vi "获取关键参数.vi"(8 "error in (no error)":errorcluster caption="错误输入（无错误）", 9 "量程":u16, 10 "flowid":u16, 11 "id":i32) -> (0 "error out":errorcluster caption="错误输出")   [LabVIEW 2016, in "斯坦道总氮V2.lvlib"]
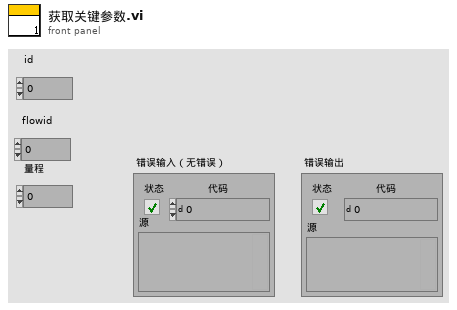
[diagram p1: front panel]
types:
  T1 = cluster{"运行模式":enum16{"维护模式", "常规模式", "应急模式", "质控模式"}, "质控频次":enum16{"关闭", "每天", "星期一", "星期二", "星期三", "星期四", "星期五", "星期六", "星期日"}, "空白核查时间":u16, "跨度核查时间":u16, "测量间隔":dbl}
  T2 = cluster{"标液浓度1":dbl, "测量吸光度1":dbl, "样品1启用":bool, "标液浓度2":dbl, "测量吸光度2":dbl, "样品2启用":bool, "标液浓度3":dbl, "测量吸光度3":dbl, "样品3启用":bool, "标液浓度4":dbl, "测量吸光度4":dbl, "样品4启用":bool, "标液浓度5":dbl, "测量吸光度5":dbl, "样品5启用":bool, "模型":enum32{"线性", "多项式"}, "精度":dbl, "XY图":cluster{"X Values":dbl[], "Y Values":dbl[]}[], "拟合公式":string, "r^2":dbl, "标样一校准时间":timestamp, "标样二校准时间":timestamp, "标样三校准时间":timestamp, "标样四校准时间":timestamp, "标样五校准时间":timestamp, "二次方程":cluster{"c":dbl, "x":dbl, "x^2":dbl}, "标定时间":timestamp}
  T3 = cluster{"精度":dbl, "检出限":dbl, "量程上限":dbl, "量程下限":dbl}
  T4 = cluster{"总磷":dbl, "总氮":dbl, "氨氮":dbl, "磷酸盐":dbl, "硝氮":dbl, "亚硝氮":dbl, "硅酸盐":dbl, "硫化物":dbl, "COD":dbl}
  T5 = cluster{"标液浓度1":dbl, "测量吸光度1":dbl, "样品1启用":bool, "标液浓度2":dbl, "测量吸光度2":dbl, "样品2启用":bool, "标液浓度3":dbl, "测量吸光度3":dbl, "样品3启用":bool, "标液浓度4":dbl, "测量吸光度4":dbl, "样品4启用":bool, "标液浓度5":dbl, "测量吸光度5":dbl, "样品5启用":bool, "模型":enum32{"线性", "多项式"}, "精度":dbl, "XY图":cluster{"X Values":dbl[], "Y Values":dbl[]}[], "拟合公式":string, "r^2":dbl, "标样一校准时间":timestamp, "标样二校准时间":timestamp, "标样三校准时间":timestamp, "标样四校准时间":timestamp, "标样五校准时间":timestamp, "二次方程":cluster{"c":dbl, "x":dbl, "x^2":dbl}, "标定时间":timestamp}[]
  T6 = typedef "斯坦道总氮V2.lvlib/关键参数.ctl" = cluster{"测量量程":sgl, "测量检出限":sgl, "测量精度":sgl, "测量间隔":sgl, "消解温度":sgl, "消解时长":sgl, "三项式系数":sgl, "二次多项式系数":sgl, "曲线斜率":sgl, "曲线截距":sgl, "线性相关系数":sgl, "空白校准时间":timestamp, "标样校准时间":timestamp, "测量信号值":sgl, "稀释倍数":sgl, "空白标定系数":sgl, "量程系数":sgl}
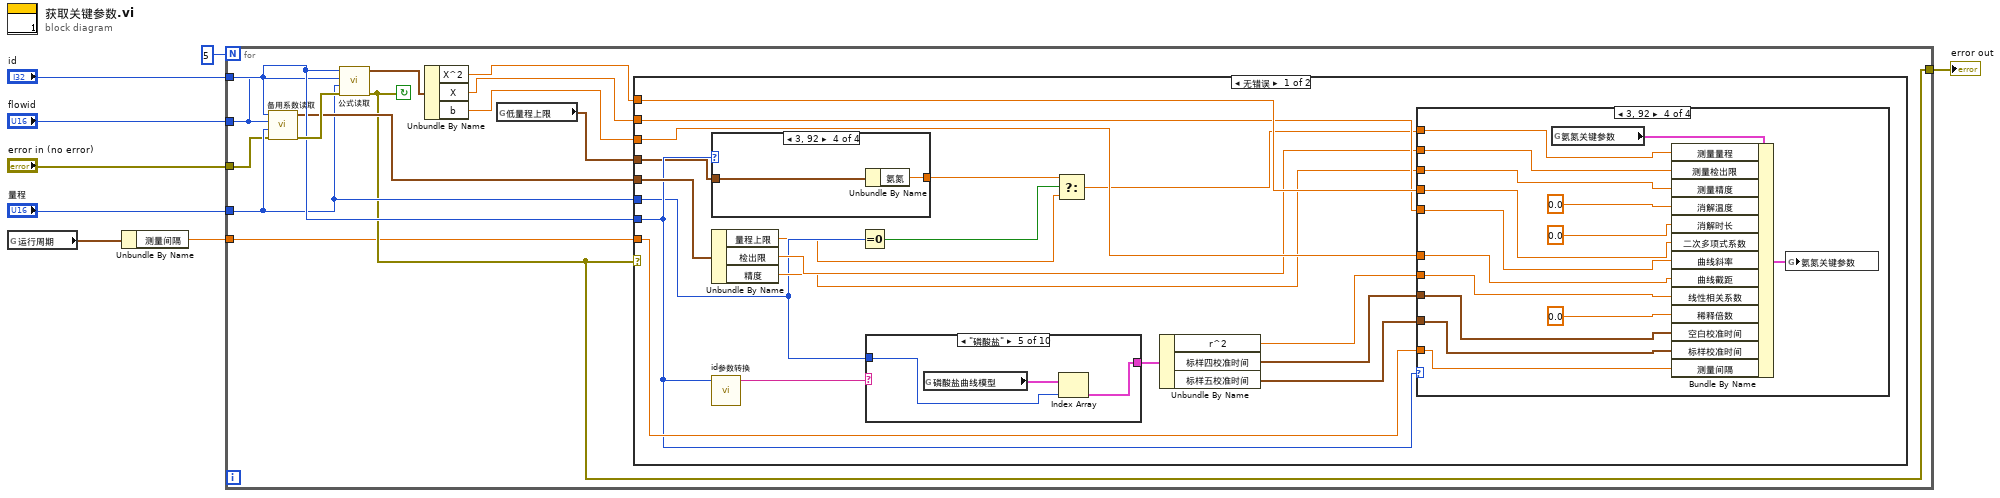
[diagram p0: block diagram]
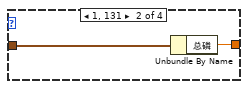
[diagram p3: hidden frame]
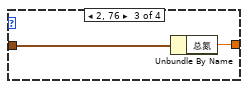
[diagram p4: hidden frame]
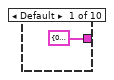
[diagram p5: hidden frame]
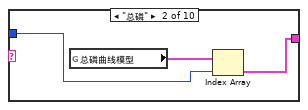
[diagram p6: hidden frame]
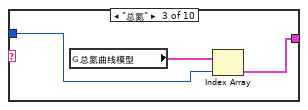
[diagram p7: hidden frame]
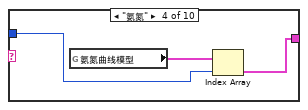
[diagram p8: hidden frame]
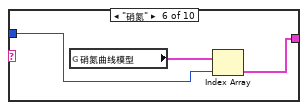
[diagram p9: hidden frame]
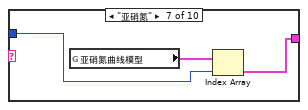
[diagram p10: hidden frame]
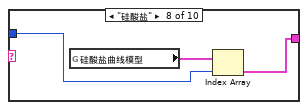
[diagram p11: hidden frame]
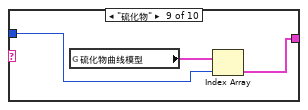
[diagram p12: hidden frame]
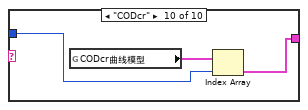
[diagram p13: hidden frame]
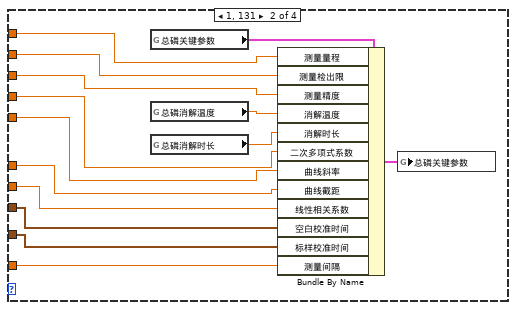
[diagram p15: hidden frame]
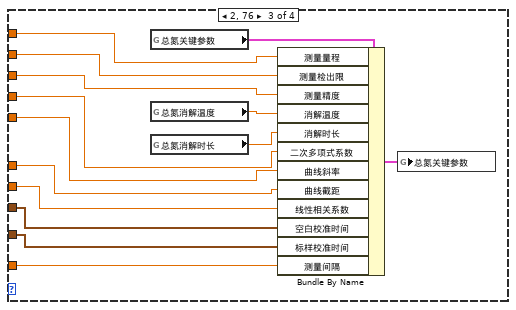
[diagram p16: hidden frame]
diagram:
  n1 = global read "总磷总氮断电保存全局变量.vi" "运行周期"() -> (w2:T1)
  n2 = Unbundle By Name(w2) -> ("测量间隔"=w1:dbl)
  n3 = for {
    N: 5 -> [_]
    tunnel: "量程" -> [w14]
    tunnel: "flowid" -> [w13]
    tunnel: "id" -> [w16]
    tunnel: "error in (no error)" -> [w12]
    tunnel: [w11] -> w3
    tunnel: w1 -> [w10]
    stop <- w11 continue-if-true
    n4 = call "备用系数读取.vi"("error in (no error)"=w12, "量程下拉列表"=w14, "测量模式"=w13, "参数下拉列表"=w16) -> ("error out"=w17:errorcluster, "备用系数"=w15:T3)  [unwired: 6 in]
    n5 = call "公式读取.vi"("error in (no error)"=w17, "量程下拉列表"=w14, "测量模式"=w13, "参数下拉列表"=w16) -> ("error out"=w11:errorcluster, "公式"=w21:cluster{"X^2":dbl, "X":dbl, "b":dbl})  [unwired: 6 in]
    n6 = Unbundle By Name(w21) -> ("X^2"=w20:dbl, "X"=w19:dbl, "b"=w18:dbl)
    n7 = global read "总磷总氮断电保存全局变量.vi" "低量程上限"() -> (w9:T4)
    n8 = case shown="无错误" w11 {
      tunnel: w20 -> [w40 _]
      tunnel: w19 -> [w39 _]
      tunnel: w18 -> [w38 _]
      tunnel: w16 -> [w28 _]
      tunnel: w14 -> [w26 _]
      tunnel: w15 -> [w32 _]
      tunnel: w10 -> [w29 _]
      tunnel: w9 -> [w27 _]
      frame No Error {
        n9 = case shown="3, 92" w28 {
          tunnel: w27 -> [_ w42 w44 w46]
          tunnel: [_ w41 w43 w45] -> w24
          frame 0, Default {
          }
          frame 1, 131 {
            n10 = Unbundle By Name(w42) -> ("总磷"=w41:dbl)
          }
          frame 2, 76 {
            n11 = Unbundle By Name(w44) -> ("总氮"=w43:dbl)
          }
          frame 3, 92 {
            n12 = Unbundle By Name(w46) -> ("氨氮"=w45:dbl)
          }
        }
        n13 = Unbundle By Name(w32) -> ("量程上限"=w23:dbl, "检出限"=w31:dbl, "精度"=w30:dbl)
        n14 = call "id参数转换.vi"("id"=w28) -> ("table输出"=w37:string)  [unwired: 9 in, 1 out]
        n15 = Equal To 0?(x=w26) -> (x = 0?=w25:bool)
        n16 = case shown="\"磷酸盐\"" w37 {
          tunnel: w26 -> [_ w48 w51 w54 w57 w60 w63 w66 w69 w72]
          tunnel: [T2 {"标液浓度1"=0.0, "测量吸光度1"=0.0, "样品1启用"=FALSE, "标液浓度2"=0.0, "测量吸光度2"=0.0, "样品2启用"=FALSE, "标液浓度3"=0.0, "测量吸光度3"=0.0, "样品3启用"=FALSE, "标液浓度4"=0.0, "测量吸光度4"=0.0, "样品4启用"=FALSE, "标液浓度5"=0.0, "测量吸光度5"=0.0, "样品5启用"=FALSE, "模型"=enum."线性", "精度"=0.0, "XY图"=[], "拟合公式"="", "r^2"=0.0, "标样一校准时间"=timestamp(0 s since 1904-01-01), "标样二校准时间"=timestamp(0 s since 1904-01-01), "标样三校准时间"=timestamp(0 s since 1904-01-01), "标样四校准时间"=timestamp(0 s since 1904-01-01), "标样五校准时间"=timestamp(0 s since 1904-01-01), "二次方程"={"c"=0.0, "x"=0.0, "x^2"=0.0}, "标定时间"=timestamp(0 s since 1904-01-01)} ("总磷曲线模型") w49 w52 w55 w58 w61 w64 w67 w70 w73] -> w36
          frame Default {
          }
          frame "总磷" {
            n17 = global read "校准数据全局变量.vi" "总磷曲线模型"() -> (w50:T5)
            n18 = Index Array(array=w50, index=w48) -> (element=w49:T2)
          }
          frame "总氮" {
            n19 = global read "校准数据全局变量.vi" "总氮曲线模型"() -> (w53:T5)
            n20 = Index Array(array=w53, index=w51) -> (element=w52:T2)
          }
          frame "氨氮" {
            n21 = global read "校准数据全局变量.vi" "氨氮曲线模型"() -> (w56:T5)
            n22 = Index Array(array=w56, index=w54) -> (element=w55:T2)
          }
          frame "磷酸盐" {
            n23 = global read "校准数据全局变量.vi" "磷酸盐曲线模型"() -> (w59:T5)
            n24 = Index Array(array=w59, index=w57) -> (element=w58:T2)
          }
          frame "硝氮" {
            n25 = global read "校准数据全局变量.vi" "硝氮曲线模型"() -> (w62:T5)
            n26 = Index Array(array=w62, index=w60) -> (element=w61:T2)
          }
          frame "亚硝氮" {
            n27 = global read "校准数据全局变量.vi" "亚硝氮曲线模型"() -> (w65:T5)
            n28 = Index Array(array=w65, index=w63) -> (element=w64:T2)
          }
          frame "硅酸盐" {
            n29 = global read "校准数据全局变量.vi" "硅酸盐曲线模型"() -> (w68:T5)
            n30 = Index Array(array=w68, index=w66) -> (element=w67:T2)
          }
          frame "硫化物" {
            n31 = global read "校准数据全局变量.vi" "硫化物曲线模型"() -> (w71:T5)
            n32 = Index Array(array=w71, index=w69) -> (element=w70:T2)
          }
          frame "CODcr" {
            n33 = global read "校准数据全局变量.vi" "CODcr曲线模型"() -> (w74:T5)
            n34 = Index Array(array=w74, index=w72) -> (element=w73:T2)
          }
        }
        n35 = Select(t=w24, s=w25, f=w23) -> (s? t:f=w22:dbl)
        n36 = Unbundle By Name(w36) -> ("r^2"=w35:dbl, "标样四校准时间"=w34:timestamp, "标样五校准时间"=w33:timestamp)
        n37 = case shown="3, 92" w28 {
          tunnel: w40 -> [_ w85 w99 w115]
          tunnel: w39 -> [_ w84 w98 w114]
          tunnel: w38 -> [_ w83 w97 w113]
          tunnel: w35 -> [_ w80 w96 w110]
          tunnel: w34 -> [_ w81 w95 w109]
          tunnel: w33 -> [_ w82 w94 w108]
          tunnel: w22 -> [_ w78 w93 w106]
          tunnel: w31 -> [_ w77 w92 w105]
          tunnel: w30 -> [_ w76 w91 w104]
          tunnel: w29 -> [_ w75 w89 w103]
          frame 0, Default {
          }
          frame 1, 131 {
            n38 = global read "VAR总磷总氮全局变量.vi" "总磷关键参数"() -> (w87:T6)
            n39 = global read "总磷总氮断电保存全局变量.vi" "总磷消解温度"() -> (w79:dbl)
            n40 = global read "总磷总氮断电保存全局变量.vi" "总磷消解时长"() -> (w86:dbl)
            n41 = Bundle By Name(cluster=w87, "测量量程"=w78, "测量检出限"=w77, "测量精度"=w76, "消解温度"=w79, "消解时长"=w86, "二次多项式系数"=w85, "曲线斜率"=w84, "曲线截距"=w83, "线性相关系数"=w80, "空白校准时间"=w81, "标样校准时间"=w82, "测量间隔"=w75) -> (w88:T6)
            n42 = global write "VAR总磷总氮全局变量.vi" "总磷关键参数"(w88) -> ()
          }
          frame 2, 76 {
            n43 = global read "VAR总磷总氮全局变量.vi" "总氮关键参数"() -> (w101:T6)
            n44 = global read "总磷总氮断电保存全局变量.vi" "总氮消解温度"() -> (w90:dbl)
            n45 = global read "总磷总氮断电保存全局变量.vi" "总氮消解时长"() -> (w100:dbl)
            n46 = Bundle By Name(cluster=w101, "测量量程"=w93, "测量检出限"=w92, "测量精度"=w91, "消解温度"=w90, "消解时长"=w100, "二次多项式系数"=w99, "曲线斜率"=w98, "曲线截距"=w97, "线性相关系数"=w96, "空白校准时间"=w95, "标样校准时间"=w94, "测量间隔"=w89) -> (w102:T6)
            n47 = global write "VAR总磷总氮全局变量.vi" "总氮关键参数"(w102) -> ()
          }
          frame 3, 92 {
            n48 = global read "VAR总磷总氮全局变量.vi" "氨氮关键参数"() -> (w116:T6)
            n49 = Bundle By Name(cluster=w116, "测量量程"=w106, "测量检出限"=w105, "测量精度"=w104, "消解温度"=sgl 0.0, "消解时长"=sgl 0.0, "二次多项式系数"=w115, "曲线斜率"=w114, "曲线截距"=w113, "线性相关系数"=w110, "稀释倍数"=sgl 0.0, "空白校准时间"=w109, "标样校准时间"=w108, "测量间隔"=w103) -> (w117:T6)
            n50 = global write "VAR总磷总氮全局变量.vi" "氨氮关键参数"(w117) -> ()
          }
        }
      }
      frame Error {
      }
    }
  }
  "error out" <- w3
